vi "FinalStringFormatting.vi"(7 "Decimal Notation (.)":string=".", 10 "Equals Zero?":bool, 11 "String in":string) -> (3 "String out":string)   [LabVIEW 2013, in "OpenScalar.lvlib"]
uses:
  OpenScalar.lvlib
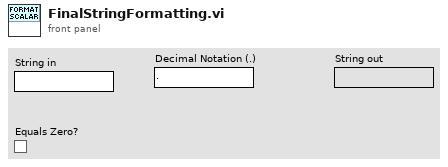
[diagram p1: front panel]
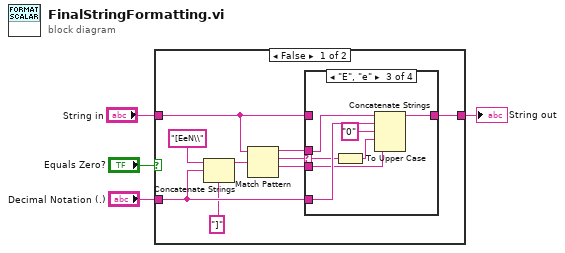
[diagram p0: block diagram]
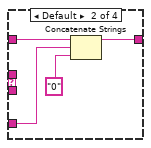
[diagram p3: hidden frame]
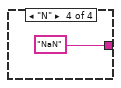
[diagram p4: hidden frame]
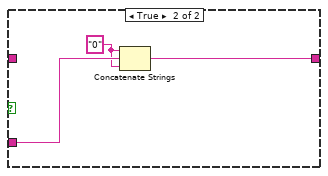
[diagram p5: hidden frame]
diagram:
  n1 = case shown="False" "Equals Zero?" {
    tunnel: [w13 w28] -> w3
    tunnel: "String in" -> [w11 _]
    tunnel: "Decimal Notation (.)" -> [w8 w29]
    frame False {
      n2 = Concatenate Strings("[EeN\\" ("string"), w8, "]" ("string")) -> (w9:string)
      n3 = Match Pattern(string=w11, regular expression=w9) -> (before substring=w7:string, match substring=w12:string, after substring=w6:string)  [unwired: 1 in, 1 out]
      n4 = case shown="\"E\", \"e\"" w12 {
        selector: w12 -> [_ _ w21 _]
        tunnel: w11 -> [w14 w17 _ _]
        tunnel: [w14 w18 w25 "NaN" ("string")] -> w13
        tunnel: w8 -> [_ w15 w23 _]
        tunnel: w7 -> [_ _ w22 _]
        tunnel: w6 -> [_ _ w20 _]
        frame ",", "." {
          # "Found a\ndecimal separator\n(before exponent)\nor NaN"
        }
        frame Default {
          n5 = Concatenate Strings(w17, w15, "0" ("regular expression")) -> (w18:string)
        }
        frame "E", "e" {
          n6 = To Upper Case(1:w21) -> (0:w19:string)
          n7 = Concatenate Strings(w22, w23, "0" ("regular expression"), w19, w20) -> (w25:string)
        }
        frame "N" {
        }
      }
    }
    frame True {
      w27 = "0" ("regular expression")
      n8 = Concatenate Strings(w27, w29, w27) -> (w28:string)
    }
  }
  "String out" <- w3
